vi "Init.vi"(8 "error in (no error)":errorcluster, 10 "Params":variant, 11 "NI DMM in":refnum<class "NI DMM.lvclass">) -> (0 "error out":errorcluster, 3 "NI DMM out":refnum<class "NI DMM.lvclass">)   [LabVIEW 2020, in "NI DMM.lvlib" / "NI DMM.lvclass"]
uses:
  NI DMM.lvclass
  NI DMM.lvclass/NI DMM.ctl
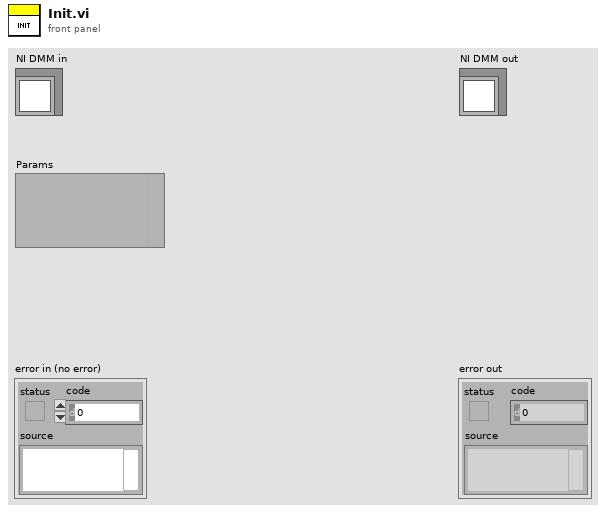
[diagram p1: front panel]
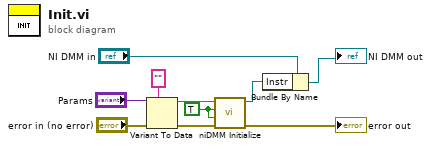
[diagram p0: block diagram]
diagram:
  w4 = TRUE ("ID Query")
  n1 = Variant To Data(error in="error in (no error)", type="", Variant="Params") -> (data=w5:string, error out=w3:errorcluster)
  n2 = call <instrlib>:"niDMM Initialize.vi"("error in (no error)"=w3, "Reset"=w4, "ID Query"=w4, "Instrument Descriptor"=w5) -> ("error out"=→"error out":errorcluster, "instrument handle out"=w2:refnum<k15>)  [unwired: 6 in]
  n3 = Bundle By Name(cluster="NI DMM in", "Instr"=w2) -> (→"NI DMM out":refnum<class "NI DMM.lvclass">)
